vi "Initialise.vi"(8 "error in (no error)":errorcluster, 11 "Actor in":refnum<class "Process Input View.lvclass">) -> (0 "error out":errorcluster, 3 "Actor out":refnum<class "Process Input View.lvclass">, 5 "Observers":cluster{"Actor":refnum<event-registration>})   [LabVIEW 2015, in "Process Input View.lvclass"]
uses:
  Process Input View.lvclass
  Re-use Libraries/Utility/Utility.lvlib
  Re-use Libraries/Minimal Actor Framework/Messaging/Message/Message.lvclass
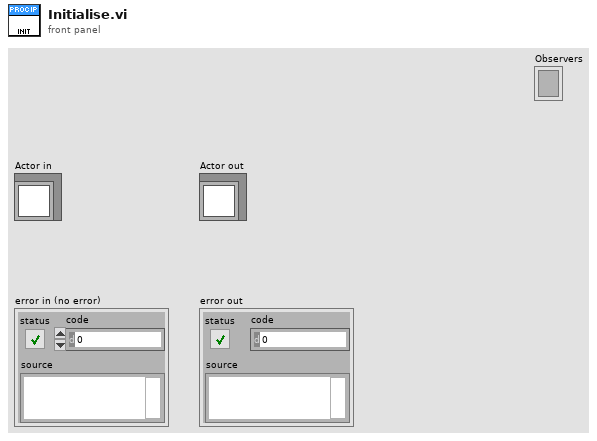
[diagram p1: front panel]
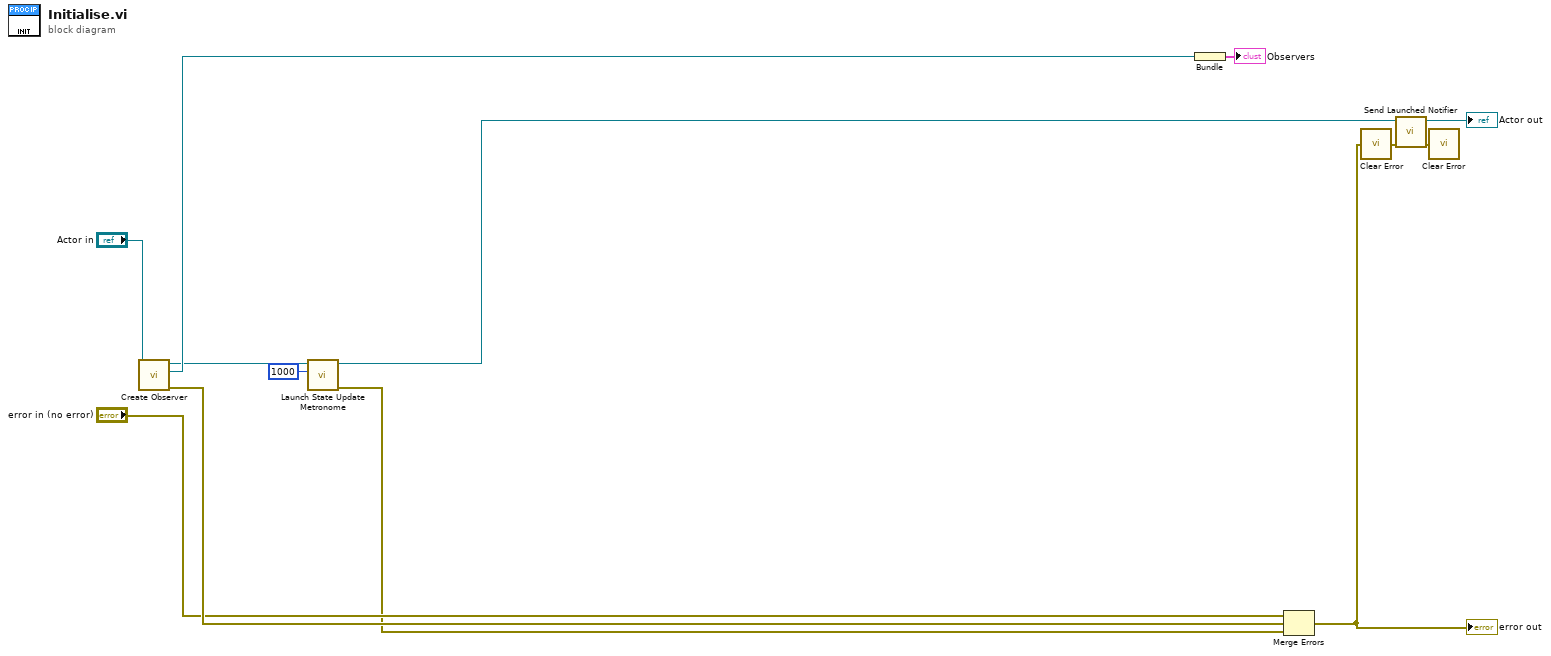
[diagram p0: block diagram]
diagram:
  n1 = call-dynamic "Create Observer.vi"("Actor in"="Actor in") -> ("error out"=w11:errorcluster, "Actor"=w6:refnum<event-registration>, "Actor out"=w4:refnum<class "Process Input View.lvclass">)  [unwired: 8 in]
  n2 = call-dynamic "Launch State Update Metronome.vi"("Status Update Period [1000 ms]"=1000, "Actor in"=w4) -> ("error out"=w1:errorcluster, "Actor out"=w3:refnum<class "Process Input View.lvclass">)  [unwired: 8 in]
  n3 = Bundle("Actor"=w6) -> (→"Observers":cluster{"Actor":refnum<event-registration>})  [unwired: 1 in]
  n4 = Merge Errors("error in (no error)", w11, w1) -> (w10:errorcluster)
  "error out" <- w10
  n5 = call "Clear Error.vi"("error in (no error)"=w10) -> ("error out"=w9:errorcluster)
  n6 = call-dynamic "Send Launched Notifier.vi"("error in (no error)"=w9, "Actor in"=w3) -> ("error out"=w8:errorcluster, "Actor out"=→"Actor out":refnum<class "Process Input View.lvclass">)  [unwired: 8 in]
  n7 = call "Clear Error.vi"("error in (no error)"=w8) -> ()  [unwired: 1 out]
